vi "Simulated VeriStand Engine.Interface.Create.vi"(8 "error in (no error)":errorcluster, 11 "Simulated VeriStand Engine Interface in":refnum<class "Simulated VeriStand Engine.Interface.lvclass">) -> (0 "error out":errorcluster, 3 "Simulated VeriStand Engine Interface out":refnum<class "Simulated VeriStand Engine.Interface.lvclass">)   [LabVIEW 2016, in "Simulated VeriStand Engine.Interface.lvclass"]
uses:
  Simulated VeriStand Engine.Interface.lvclass
  Simulated VeriStand Engine.Interface.lvclass/Simulated VeriStand Engine.Interface.ctl
  Source/Submodules/Memory/Source/Classes/Internal/Memory.Pointer.Internal.New.vi
  Accessors/Simulated VeriStand Engine.Interface.Set Status Pointers.vi
  Accessors/Simulated VeriStand Engine.Interface.Set Control Pointers.vi
  Source/Submodules/Memory/Source/Classes/Internal/Memory.Pointer.Internal.Allocate.vi
  Source/Submodules/Memory/Source/Classes/Internal/Memory.Pointer.Internal.lvclass
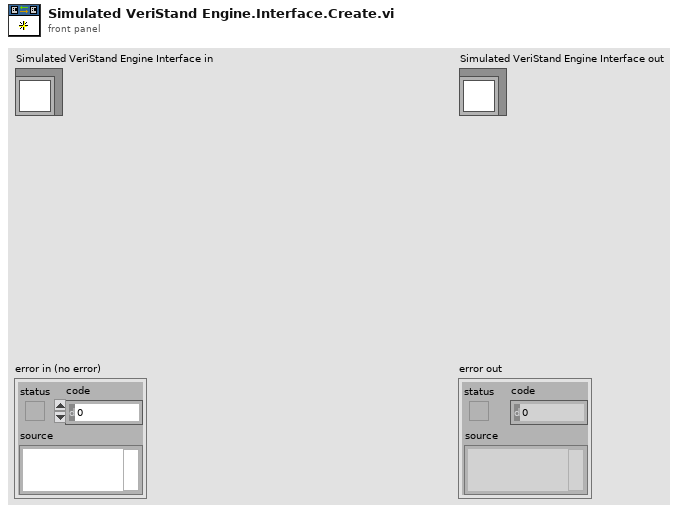
[diagram p1: front panel]
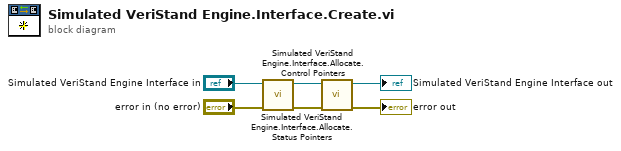
[diagram p0: block diagram]
diagram:
  n1 = call "Simulated VeriStand Engine.Interface.Allocate.Control Pointers.vi"("error in (no error)"="error in (no error)", "Simulated VeriStand Engine Interface in"="Simulated VeriStand Engine Interface in") -> ("error out"=w3:errorcluster, "Simulated VeriStand Engine Interface out"=w4:refnum<class "Simulated VeriStand Engine.Interface.lvclass">)  [unwired: 8 in]
  n2 = call "Simulated VeriStand Engine.Interface.Allocate.Status Pointers.vi"("error in (no error)"=w3, "Simulated VeriStand Engine Interface in"=w4) -> ("error out"=→"error out":errorcluster, "Simulated VeriStand Engine Interface out"=→"Simulated VeriStand Engine Interface out":refnum<class "Simulated VeriStand Engine.Interface.lvclass">)  [unwired: 8 in]
